vi "USB2XXXADS1256.vi"() -> ()   [LabVIEW 2010]
uses:
  PublicFiles/usb_device/USB2XXX.dll
panel:
  in  "Stop":bool
  in  "pConfig":T1
  out "mVp-p":dbl
  out "DC":dbl
  out "RMS":dbl
  out "Waveform Chart":dbl(graph)
  in  "Channel Index":i8(ring) items=["SPI1_CS0", "SPI2_CS0"]
  in  "Device Index":i32(ring) items=["0", "1", "2", "3", "4", "5"]
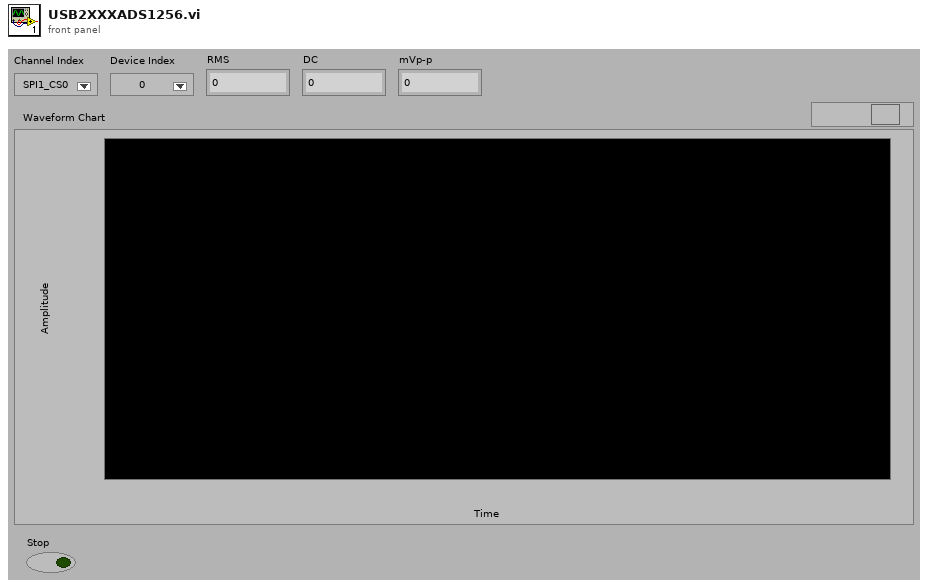
[diagram p1: front panel]
types:
  T1 = cluster{"SampleRate":u16, "PGA":u8, "BufferEn":u8, "SampleMode":u32}
  T2 = enum16{"Init ADS1256", "Read Data", "Close", "Stop Read"}
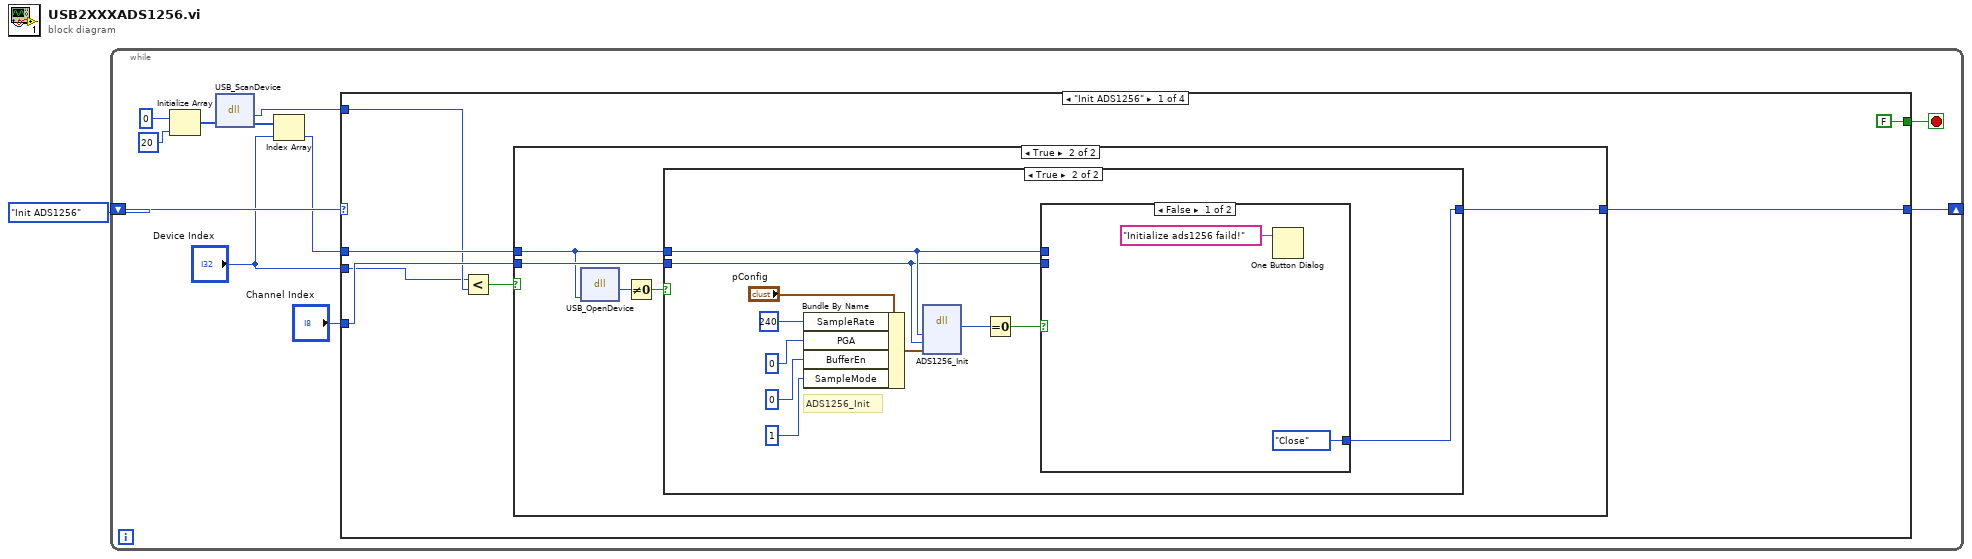
[diagram p0: block diagram]
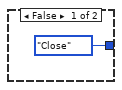
[diagram p2: hidden frame]
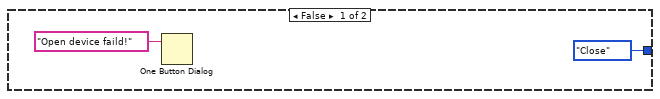
[diagram p3: hidden frame]
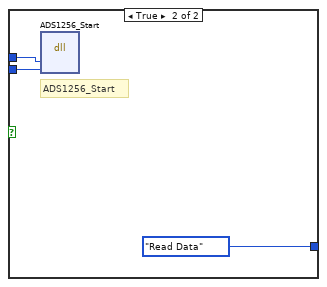
[diagram p4: hidden frame]
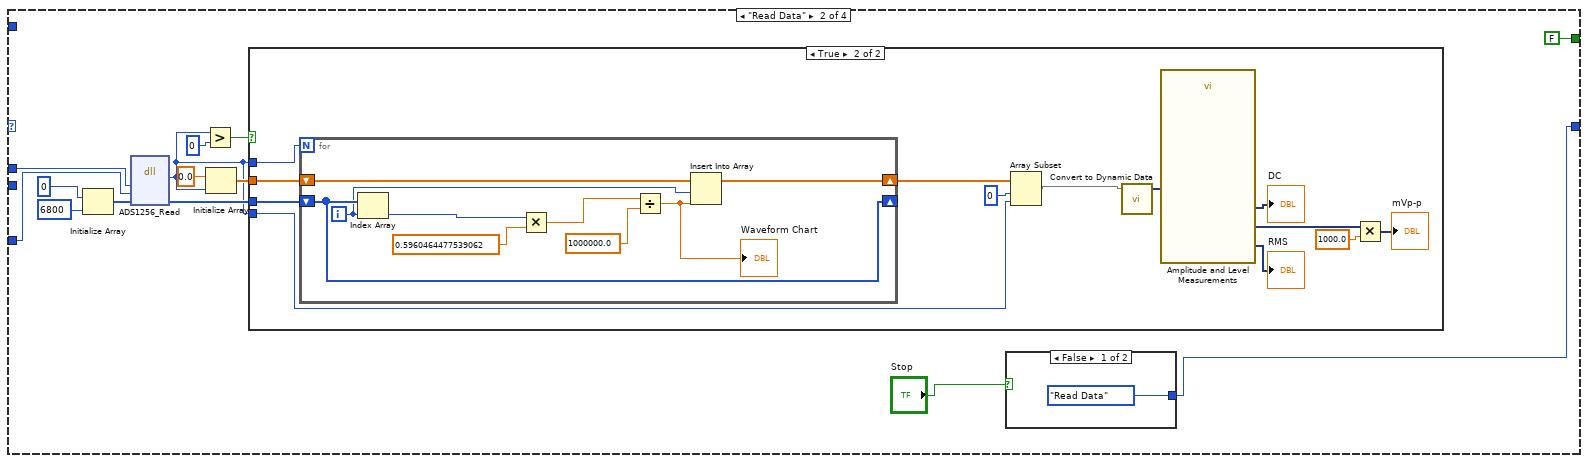
[diagram p5: hidden frame]
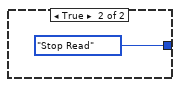
[diagram p6: hidden frame]
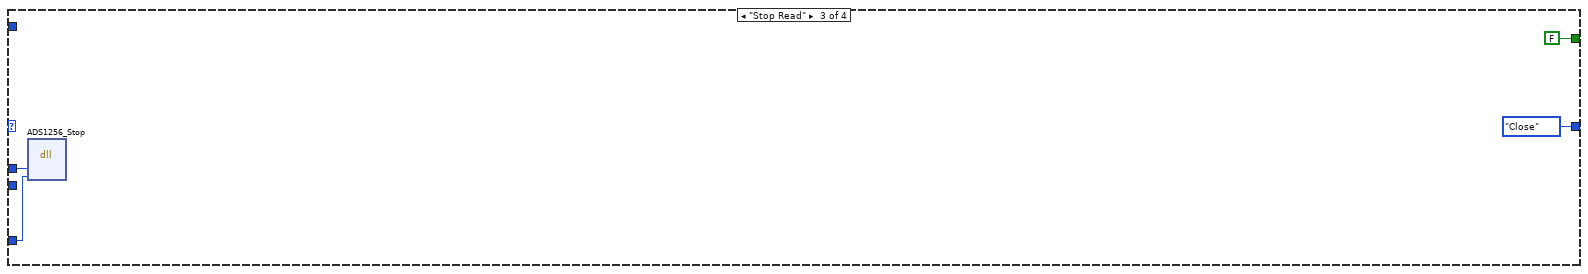
[diagram p8: hidden frame]
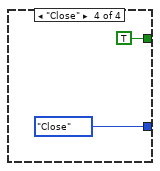
[diagram p9: hidden frame]
diagram:
  n1 = while {
    shift-right: [w11] -> _
    shift-left: T2."Init ADS1256" ("Enum") -> [w12]
    stop <- w10 stop-if-true
    n2 = Initialize Array(0, 20 ("dimension size")) -> (w8:i32[])
    n3 = dll-call lib="G:/OtherWork/USB2XXX_Example/trunk/Labview/PublicFiles/usb_device/USB2XXX.*" fn="USB_ScanDevice"("pDevNum"=w8) -> ("return type"=w3:i32, "pDevNum"=w5:i32[])  [unwired: 3 in, 2 out]
    n4 = Index Array(array=w5, index="Device Index") -> (element=w4:i32)
    n5 = case shown="\"Init ADS1256\"" w12 {
      tunnel: [w18 w44 T2."Close" ("Enum") T2."Close" ("Enum")] -> w11
      tunnel: w4 -> [w15 w50 w84 _]
      tunnel: "Channel Index" -> [w17 w49 w83 _]
      tunnel: [FALSE FALSE FALSE TRUE] -> w10
      tunnel: w3 -> [w14 _ _ _]
      tunnel: "Device Index" -> [w13 _ _ _]
      frame "Init ADS1256" {
        n6 = Less?(x=w13, y=w14) -> (x < y?=w19:bool)
        n7 = case shown="True" w19 {
          tunnel: w15 -> [_ w21]
          tunnel: w17 -> [_ w23]
          tunnel: [enum16{"Init ADS1256", "Read Data", "Close"}."Close" ("Enum") w22] -> w18
          frame False {
          }
          frame True {
            n8 = dll-call lib="G:/OtherWork/USB2XXX_Example/trunk/Labview/PublicFiles/usb_device/USB2XXX.*" fn="USB_OpenDevice"("DevIndex"=w21) -> (w25:u8)  [unwired: 4 in, 2 out]
            n9 = Not Equal To 0?(x=w25) -> (x != 0?=w24:bool)
            n10 = case shown="True" w24 {
              tunnel: w23 -> [_ w28]
              tunnel: w21 -> [_ w29]
              tunnel: [enum16{"Init ADS1256", "Read Data", "Close"}."Close" ("Enum") w37] -> w22
              frame False {
                n11 = One Button Dialog(message="Open device faild!") -> ()  [unwired: 1 in, 1 out]
              }
              frame True {
                # "ADS1256_Init"
                n12 = Bundle By Name(cluster="pConfig", "SampleRate"=u16 240, "PGA"=u8 0, "BufferEn"=u8 0, "SampleMode"=u32 1) -> (w35:T1)
                n13 = dll-call lib="G:/OtherWork/USB2XXX_Example/trunk/Labview/PublicFiles/usb_device/USB2XXX.*" fn="ADS1256_Init"("DevIndex"=w29, "Channel"=w28, "pConfig"=w35) -> (w30:i32)  [unwired: 6 in, 2 out]
                n14 = Equal To 0?(x=w30) -> (x = 0?=w38:bool)
                n15 = case shown="False" w38 {
                  tunnel: [enum16{"Init ADS1256", "Read Data", "Close"}."Close" ("Enum") enum16{"Init ADS1256", "Read Data", "Close"}."Read Data" ("Enum")] -> w37
                  tunnel: w29 -> [_ w42]
                  tunnel: w28 -> [_ w41]
                  frame False {
                    n16 = One Button Dialog(message="Initialize ads1256 faild!") -> ()  [unwired: 1 in, 1 out]
                  }
                  frame True {
                    # "ADS1256_Start"
                    n17 = dll-call lib="G:/OtherWork/USB2XXX_Example/trunk/Labview/PublicFiles/usb_device/USB2XXX.*" fn="ADS1256_Start"("DevIndex"=w42, "Channel"=w41) -> ()  [unwired: 6 in, 2 out]
                  }
                }
              }
            }
          }
        }
      }
      frame "Read Data" {
        n18 = Initialize Array(0 ("element"), 6800 ("dimension size")) -> (w53:i32[])
        n19 = dll-call lib="G:/OtherWork/USB2XXX_Example/trunk/Labview/PublicFiles/usb_device/USB2XXX.*" fn="ADS1256_Read"("DevIndex"=w50, "Channel"=w49, "pData"=w53) -> (w46:i32, "pData"=w47:i32[])  [unwired: 5 in, 2 out]
        n20 = Greater?(x=w46, y=0) -> (0:w56:bool)
        n21 = Initialize Array(0.0 ("element"), w46) -> (w54:dbl[])
        n22 = case shown="True" w56 {
          tunnel: w47 -> [_ w72]
          tunnel: w54 -> [_ w68]
          tunnel: w46 -> [_ w66]
          tunnel: w46 -> [_ w62]
          frame False {
          }
          frame True {
            n23 = for {
              N: w62 -> [_]
              shift-right: [w74] -> _
              shift-left: w72 -> [w74]
              shift-right: [w76] -> w61
              shift-left: w68 -> [w77]
              i -> [w73]
              n24 = Index Array(array=w74, index=w73) -> (element=w75:i32)
              n25 = Multiply(x=w75, y=0.5960464477539062) -> (x*y=w80:dbl)
              n26 = Divide(x=w80, y=1000000.0) -> (x/y=w78:dbl)
              "Waveform Chart" <- w78
              n27 = Insert Into Array(array=w77, index=w73, new element=w78) -> (w76:dbl[])
            }
            n28 = Array Subset(array=w61, index=0, length=w66) -> (w60:dbl[])
            n29 = call "Convert to Dynamic Data"("Array"=w60) -> ("Dynamic Data Type"=w71:dynamicdata)  [unwired: 3 in]
            n30 = call "Amplitude and Level Measurements"("Signals"=w71) -> ("Mean (DC)"=→"DC":dynamicdata, "RMS"=→"RMS":dynamicdata, "Peak to Peak"=w65:dynamicdata)  [unwired: 11 in, 1 out]
            n31 = Multiply(x=w65, y=1000.0) -> (x*y=→"mVp-p":dynamicdata)
          }
        }
        n32 = case shown="False" "Stop" {
          tunnel: [T2."Read Data" ("Enum") T2."Stop Read" ("Enum")] -> w44
          frame False {
          }
          frame True {
          }
        }
      }
      frame "Stop Read" {
        n33 = dll-call lib="G:/OtherWork/USB2XXX_Example/trunk/Labview/PublicFiles/usb_device/USB2XXX.*" fn="ADS1256_Stop"("DevIndex"=w84, "Channel"=w83) -> ()  [unwired: 6 in, 2 out]
      }
      frame "Close" {
      }
    }
  }
